vi "MCU_Flashing.vi"(8 "error in (no error)":errorcluster) -> (0 "error in (out)":errorcluster)   [LabVIEW 2024, in "MCU_Flashing.lvlib"]
doc: "This template is for the Queued Message Handler design pattern.\n\nThe Event Handling Loop generates messages based on user interface actions.\n\nThe Message Handling Loop processes messages generated by the Event Handling Loop, or by other messages. The messages are string values, so new messages can be added easily to the Message Cases case structure in the Message Handling Loop. Each message cluster can also provide an optional value for Message Data, which is a variant that can be converted to whatever message-specific data is required."
uses:
  MCU_Flashing.lvlib
  support/MCU_ctrl.ctl
  controls/MCU UI Data.ctl
  PrivateControls/FGV_Queue_Control.ctl
  <vilib>/Utility/error.llb/Error Cluster From Error Code.vi
  <vilib>/ErrorRing/Error Ring.xnode
  support/Message Queue/MCU Message Queue.lvlib
  support/User Event - Stop/MCU User Event - Stop.lvlib
  Launcher/Launcher_DTU.lvlib
panel:
  out "x >= 0?":bool
  in  "MCU Flashing":T1
  in  "Config":string
  in  "DUT":string
  in  "Flash":bool
  out "queue name 2":string
  out "queue name":string
  out "Display <Replace Me>":string
  in  "Init_Neoway":bool
  in  "Exit":bool
  # "These controls have associated \"Value Changed\" events configured in the Event Structure on the diagram.\n\nReplace them (and reconfigure the Event Structure) with the controls you need for your application."
  # "This template is for the Queued Message Handler design pattern.\n\nSee the block diagram for more information on how to use this template."
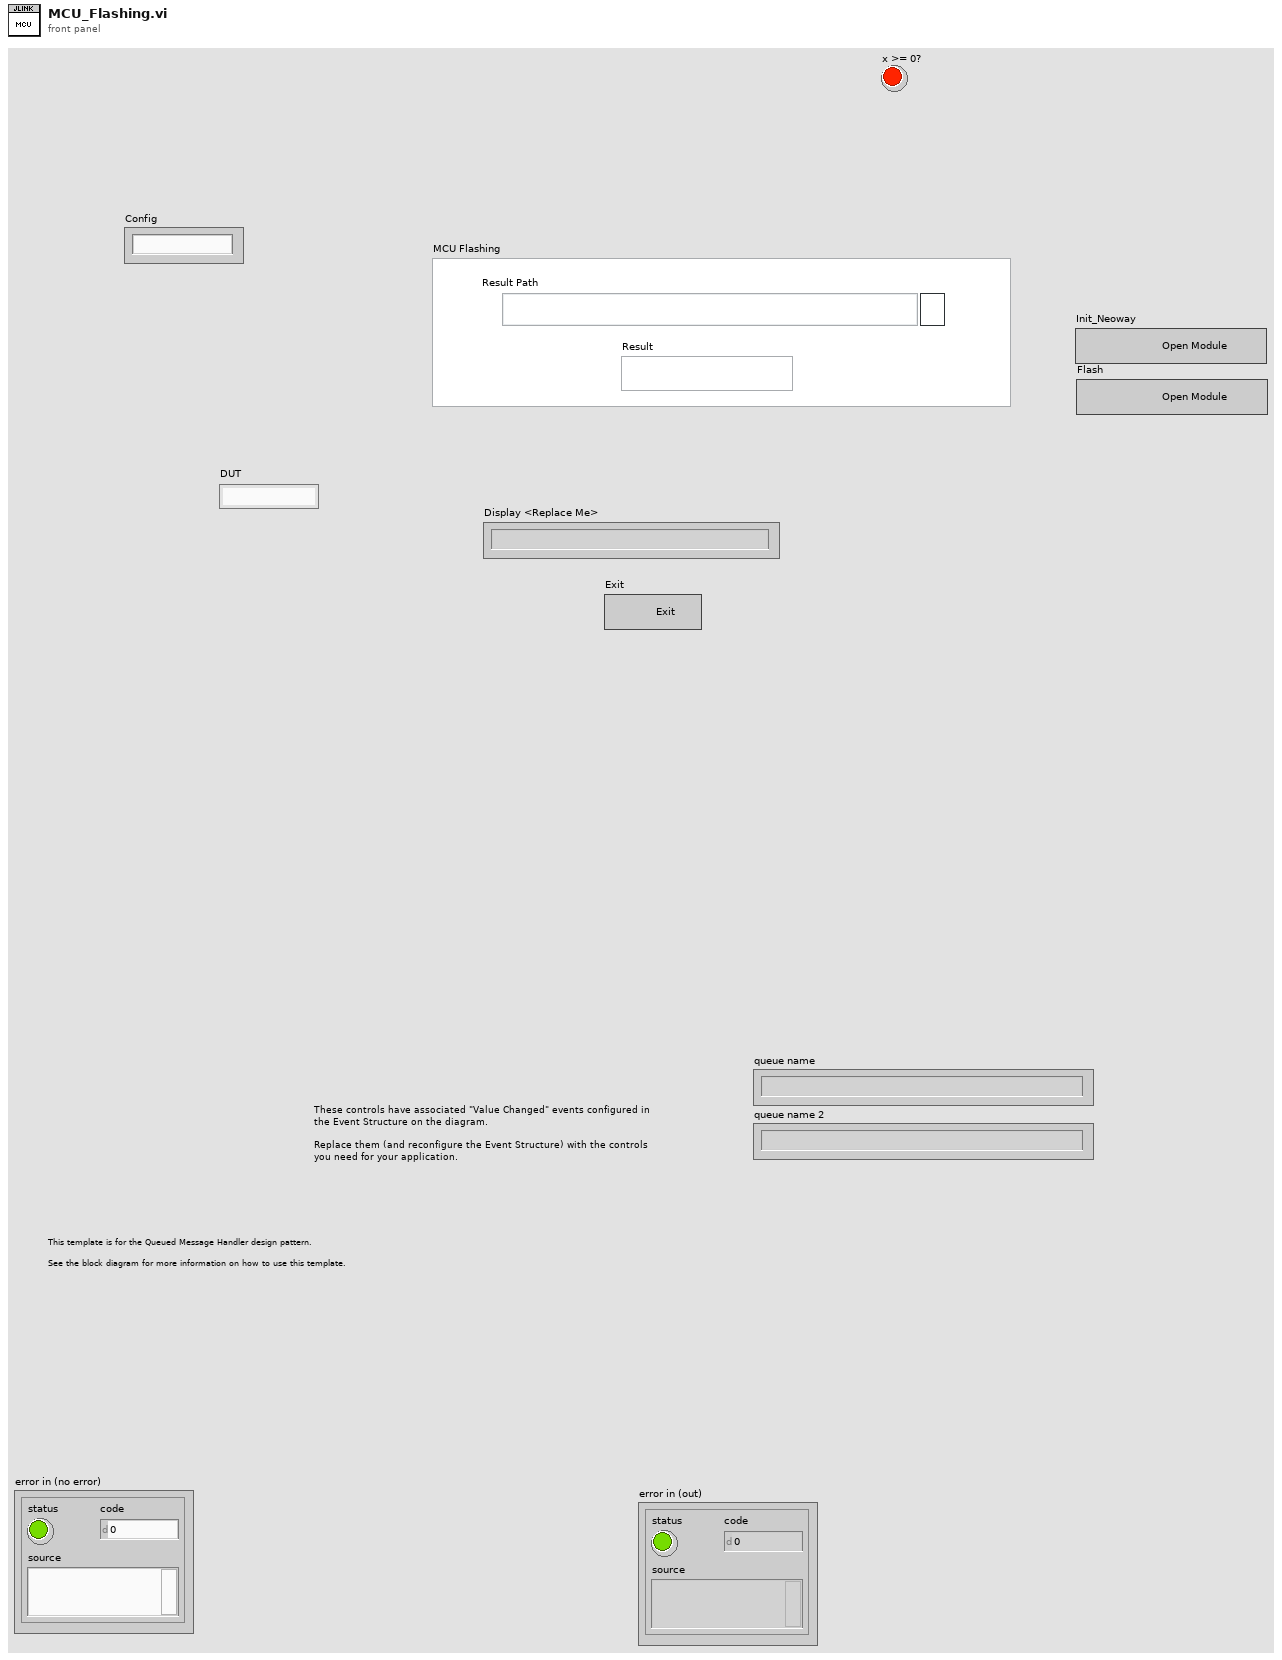
[diagram p1: front panel]
types:
  T1 = typedef "MCU_Flashing.lvlib/MCU_ctrl.ctl" = cluster{"Result Path":path, "Result":string}
  T2 = typedef "MCU_Flashing.lvlib/MCU UI Data.ctl" = cluster{"DUT":string, "Neoway_Q":refnum<queue>, "notifier out":refnum<notifier>, "Config":string, "Neoway Flashing":T1, "Bat file path":path, "Exe path":string, "Flash path":string}
  T3 = typedef "MCU_Flashing.lvlib/FGV_Queue_Control.ctl" = enum16{"Release", "Get", "Set"}
  T4 = typedef "MCU_Flashing.lvlib/MCU Message Queue.lvlib/All Message Queues.ctl" = cluster{"UI":refnum<queue>, "QSM":refnum<queue>}
  T5 = cluster{"Message":string, "Message Data":variant}
  T6 = enum16{"Read", "Write", "All_sections", "All_values", "Remove key&section"}
  T7 = enum16{"open", "replace", "create", "open or create", "replace or create", "replace or create with confirmation"}
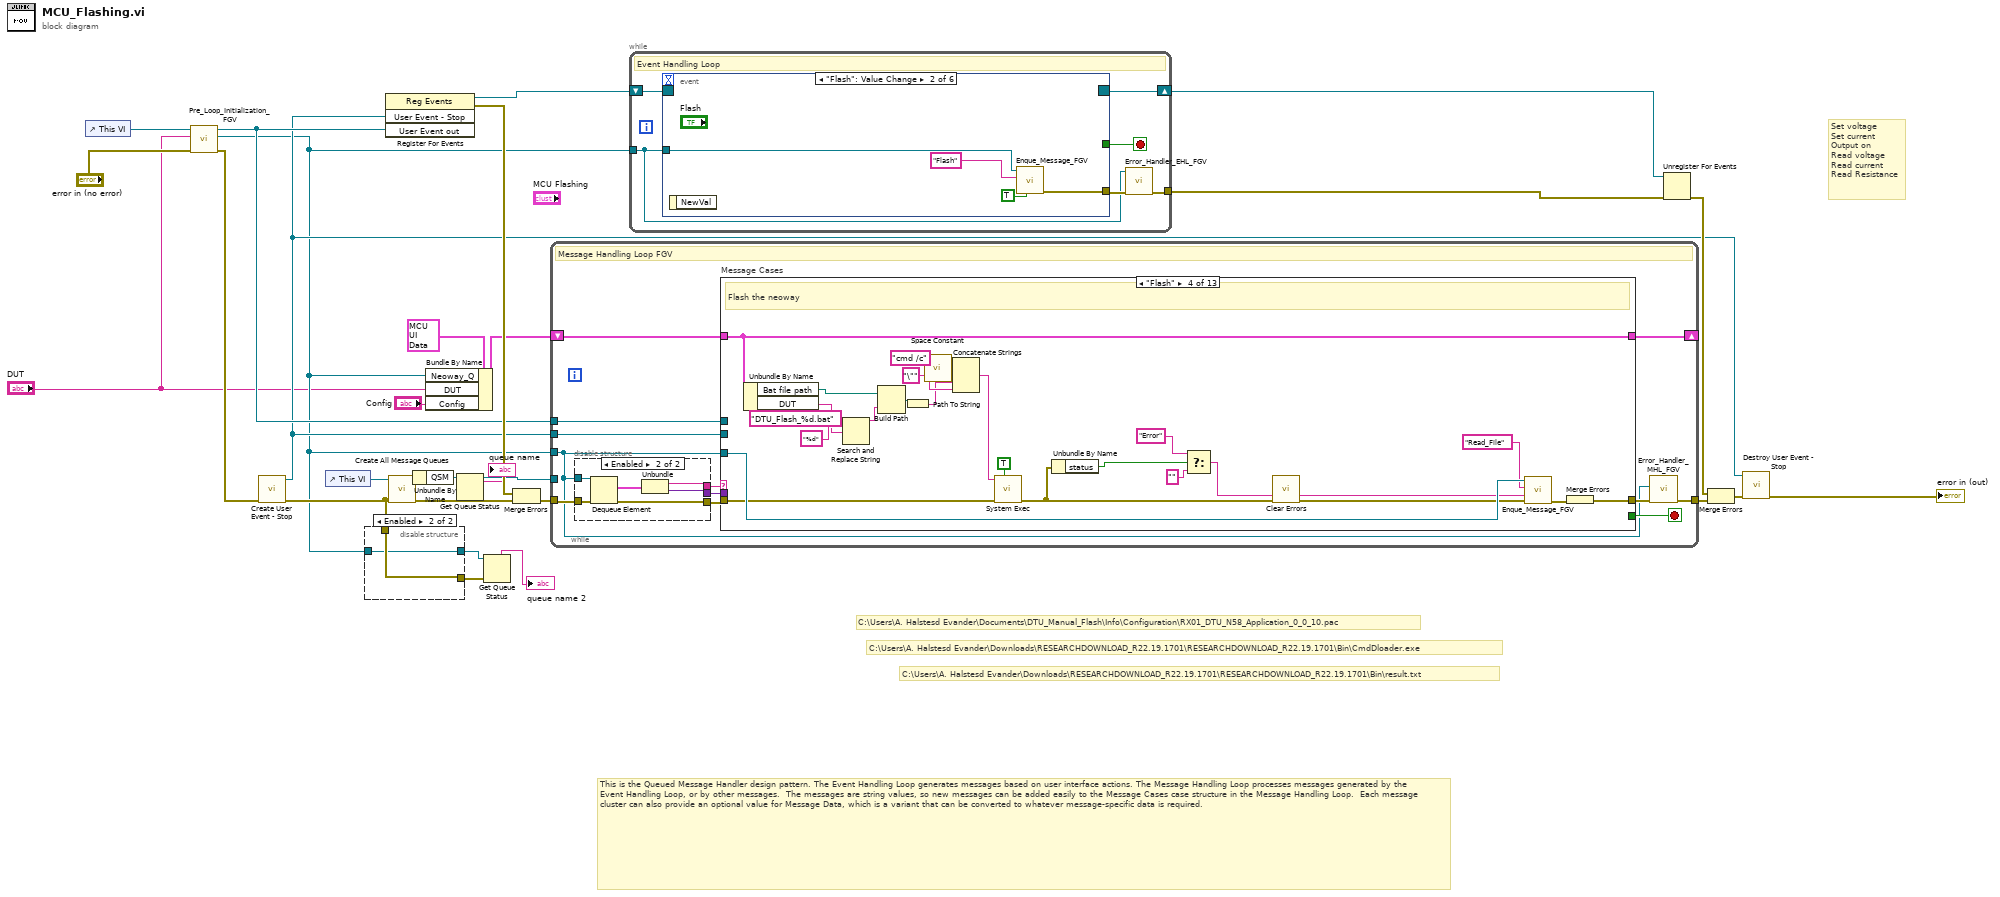
[diagram p0: block diagram]
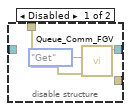
[diagram p2: hidden frame]
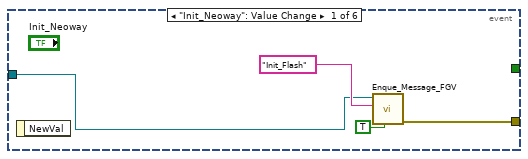
[diagram p3: hidden frame]
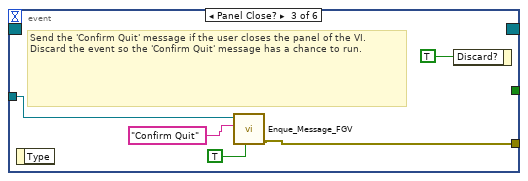
[diagram p4: hidden frame]
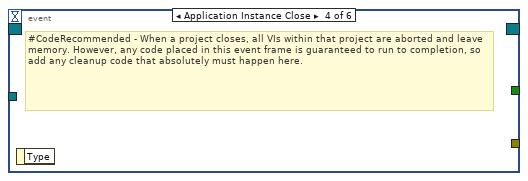
[diagram p5: hidden frame]
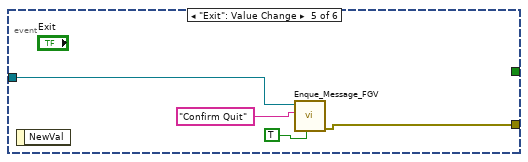
[diagram p6: hidden frame]
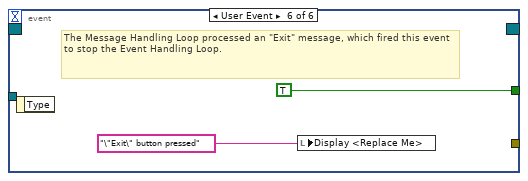
[diagram p7: hidden frame]
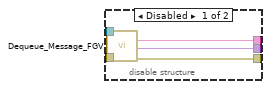
[diagram p8: hidden frame]
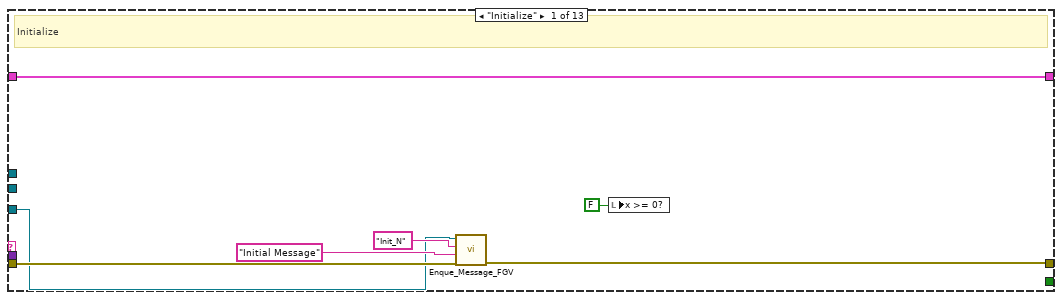
[diagram p9: hidden frame]
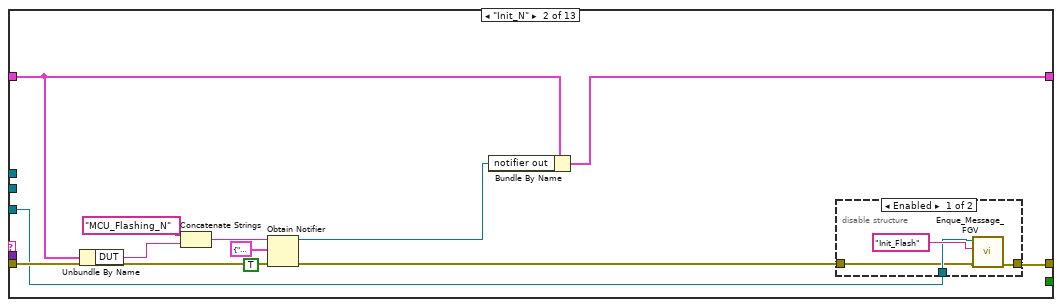
[diagram p10: hidden frame]
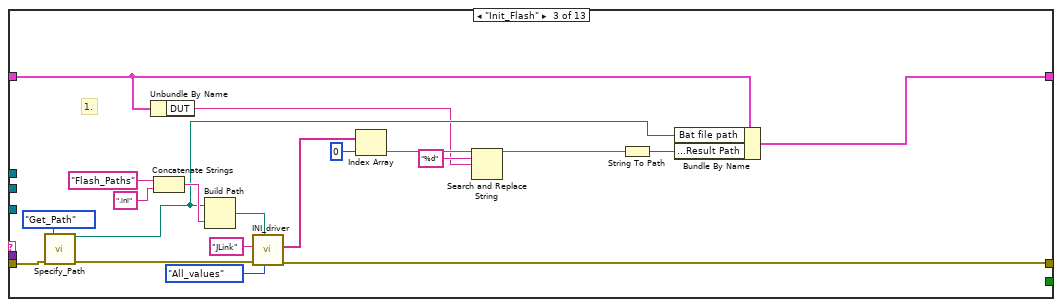
[diagram p12: hidden frame]
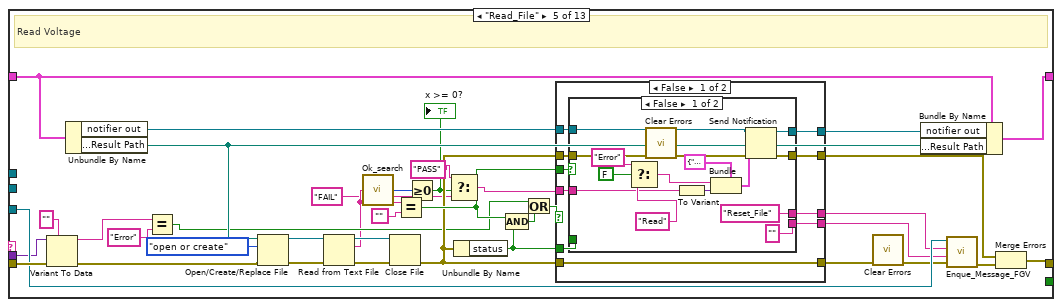
[diagram p13: hidden frame]
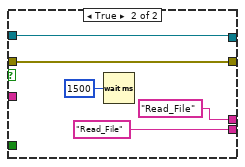
[diagram p14: hidden frame]
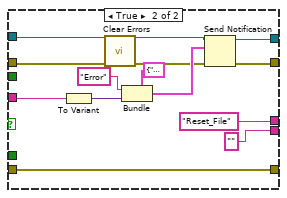
[diagram p15: hidden frame]
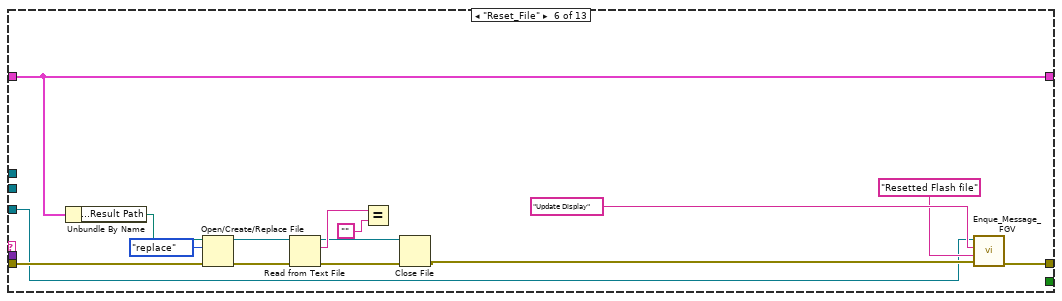
[diagram p16: hidden frame]
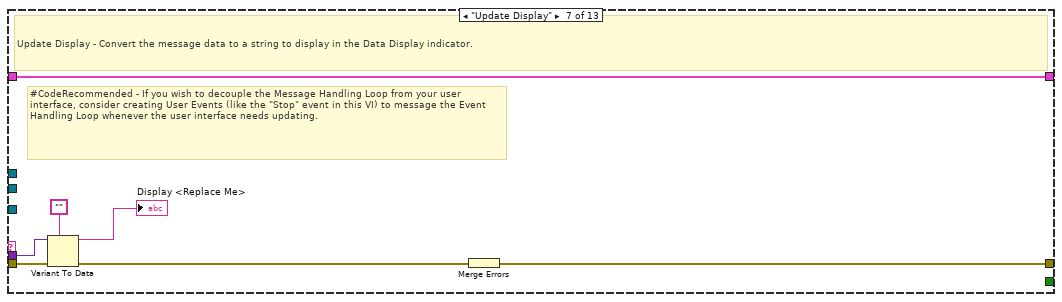
[diagram p17: hidden frame]
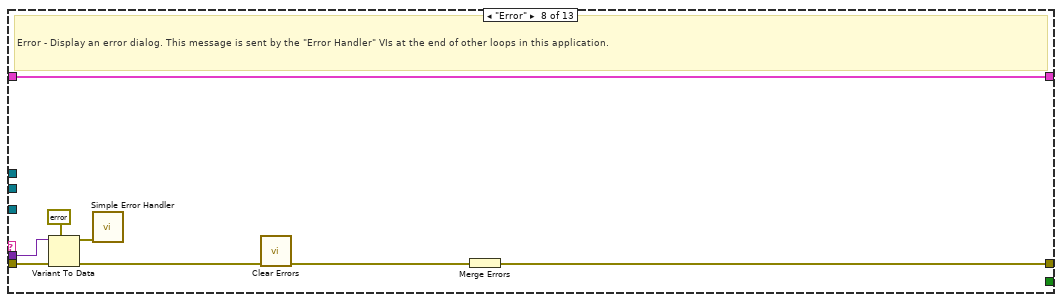
[diagram p18: hidden frame]
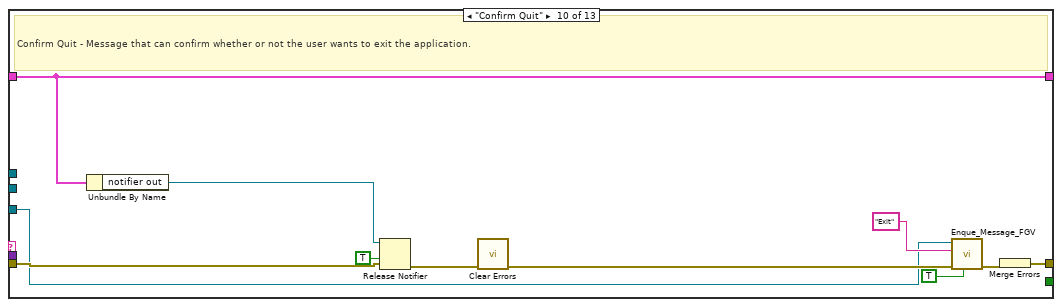
[diagram p20: hidden frame]
diagram:
  # "C:\\Users\\A. Halstesd Evander\\Downloads\\RESEARCHDOWNLOAD_R22.19.1701\\RESEARCHDOWNLOAD_R22.19.1701\\Bin\\result.txt"
  # "C:\\Users\\A. Halstesd Evander\\Downloads\\RESEARCHDOWNLOAD_R22.19.1701\\RESEARCHDOWNLOAD_R22.19.1701\\Bin\\CmdDloader.exe"
  # "C:\\Users\\A. Halstesd Evander\\Documents\\DTU_Manual_Flash\\Info\\Configuration\\RX01_DTU_N58_Application_0_0_10.pac"
  # "Set voltage\nSet current\nOutput on\nRead voltage \nRead current\nRead Resistance"
  # "This is the Queued Message Handler design pattern. The Event Handling Loop generates messages based on user interface actions. The Message Handling Loop processes messages generated by the Event Handling Loop, or by other messages.  The messages are string values, so new messages can be added easily to the Message Cases case structure in the Message Handling Loop.  Each message cluster can also provide an optional value for Message Data, which is a variant that can be converted to whatever message-specific data is required."
  n1 = control-ref of="This VI"() -> (w17:refnum<vi>)
  n2 = call "Pre_Loop_Initialization_FGV.vi"("error in (no error)"="error in (no error)", "DUT"="DUT", "VI in"=w17) -> ("error out"=w15:errorcluster, "queue out"=w3:refnum<queue>, "User Event out"=w7:refnum<user-event>)  [unwired: 6 in]
  n3 = call "Create User Event - Stop.vi"("error in (no error)"=w15) -> ("error out"=w10:errorcluster, "User Event - Stop"=w6:refnum<user-event>)  [unwired: 9 in]
  n4 = control-ref of="This VI"() -> (w13:refnum<vi>)
  n5 = disable-structure shown="Enabled" {
    disable-tunnel: w10 -> [w32 w34]
    disable-tunnel: [w30 w33] -> w9
    disable-tunnel: [_ w34] -> w5
    disable-tunnel: w3 -> [_ w33]
    frame Disabled {
      n6 = call "Queue_Comm_FGV.vi"("error in (no error)"=w32, "Enum"=FGV_Queue_Control."Get") -> ("queue Out"=w30:refnum<queue>)  [unwired: 8 in, 1 out]
    }
    frame Enabled {
    }
  }
  n7 = register-events(w6, w7) -> (reference out=w20:refnum<event-registration>, error out=w18:errorcluster)  [unwired: 2 in]
  n8 = call "Create All Message Queues.vi"("error in (no error)"=w10, "This VI"=w13) -> ("error out"=w29:errorcluster, "Message Queues out"=w28:T4)  [unwired: 8 in]
  n9 = Unbundle By Name(w28) -> ("QSM"=w26:refnum<queue>)
  n10 = Bundle By Name(cluster=T2 {"DUT"="", "Neoway_Q"=refnum, "notifier out"=refnum, "Config"="", "Neoway Flashing"={"Result Path"=path "", "Result"=""}, "Bat file path"=path "", "Exe path"="", "Flash path"=""} ("Data Cluster"), "Neoway_Q"=w3, "DUT"="DUT", "Config"="Config") -> (w4:T2)
  n11 = Get Queue Status(queue=w26) -> (queue out=w12:refnum<queue>, queue name=→"queue name":string)  [unwired: 2 in, 6 out]
  n12 = Get Queue Status(queue=w9, error in (no error)=w5) -> (queue name=→"queue name 2":string)  [unwired: 1 in, 7 out]
  n13 = Merge Errors(w18, w29) -> (w19:errorcluster)
  n14 = while {
    tunnel: w12 -> [_]
    shift-right: [w45] -> _
    shift-left: w4 -> [w46]
    tunnel: w7 -> [w43]
    tunnel: w19 -> [w42]
    tunnel: [w37] -> w27
    tunnel: w6 -> [w36]
    tunnel: w3 -> [w35]
    stop <- w44 stop-if-true
    # "Message Handling Loop FGV"
    n15 = disable-structure shown="Enabled" {
      disable-tunnel: w42 -> [w50 w56]
      disable-tunnel: [w49 w54] -> w41
      disable-tunnel: [w48 w51] -> w40
      disable-tunnel: [w47 w52] -> w39
      disable-tunnel: w35 -> [_ w55]
      frame Disabled {
        n16 = call "Dequeue_Message_FGV.vi"("error in (no error)"=w50) -> ("error out"=w49:errorcluster, "Message Data"=w48:variant, "Message"=w47:string)  [unwired: 8 in]
      }
      frame Enabled {
        n17 = Dequeue Element(queue=w55, error in (no error)=w56) -> (element=w53:T5, error out=w54:errorcluster)  [unwired: 1 in, 2 out]
        n18 = Unbundle(w53) -> ("Message"=w52:string, "Message Data"=w51:variant)
      }
    }
    n19 = case "Message Cases" shown="\"Flash\"" w39 {
      selector: w39 -> [_ _ _ _ _ _ _ _ _ _ _ _ w267]
      tunnel: w41 -> [w59 w75 w100 w121 w161 w219 w224 w234 w236 w245 w250 w258 _]
      tunnel: [w62 w64 w99 w124 w156 w206 w225 w228 w236 w247 w248 w251 w268] -> w38
      tunnel: w46 -> [w63 w73 w83 w120 w159 w218 w226 w233 w235 w242 w249 w253 w269]
      tunnel: [w63 w68 w89 w120 w158 w218 w226 w233 w235 w242 w249 w253 w269] -> w45
      tunnel: [_ _ _ _ _ _ _ _ _ _ _ TRUE _] -> w44
      tunnel: w40 -> [_ _ _ _ w155 _ w223 w232 _ _ _ w260 _]
      tunnel: w43 -> [_ _ _ _ _ _ _ _ _ _ _ w261 _]
      tunnel: w36 -> [_ _ _ _ _ _ _ _ _ _ _ w256 _]
      tunnel: w35 -> [w58 w66 _ w122 w157 w205 _ _ _ w240 _ w252 _]
      frame "Initialize" {
        # "Initialize"
        n20 = call "Enque_Message_FGV.vi"("error in (no error)"=w59, "Message Data"="Initial Message" ("Initial Message"), "Message"="Init_N", "queue in"=w58) -> ("error out"=w62:errorcluster)  [unwired: 7 in]
        n21 = local write "x >= 0?"(FALSE ("x >= 0?")) -> ()
      }
      frame "Init_N" {
        n22 = Unbundle By Name(w73) -> ("DUT"=w72:string)
        n23 = Concatenate Strings("MCU_Flashing_N", w72) -> (w71:string)
        n24 = Obtain Notifier(name (unnamed)=w71, notification data type=T5 {"Message"="", "Message Data"=variant} ("notification"), create if not found? (T)=TRUE, error in (no error)=w75) -> (notifier out=w67:refnum<notifier>, error out=w65:errorcluster)  [unwired: 1 out]
        n25 = Bundle By Name(cluster=w73, "notifier out"=w67) -> (w68:T2)
        n26 = disable-structure shown="Enabled" {
          disable-tunnel: w66 -> [w78 _]
          disable-tunnel: w65 -> [w77 w80]
          disable-tunnel: [w76 w80] -> w64
          frame Enabled {
            n27 = call "Enque_Message_FGV.vi"("error in (no error)"=w77, "Message"="Init_Flash", "queue in"=w78) -> ("error out"=w76:errorcluster)  [unwired: 8 in]
          }
          frame Disabled {
          }
        }
      }
      frame "Init_Flash" {
        # "1."
        n28 = call "Specify_Path.vi"("Path_Enum"=enum16{"Find_Path", "Get_Path"}."Get_Path", "error in (no error)"=w100) -> ("Configurations"=w86:path, "error out"=w94:errorcluster)  [unwired: 6 in, 6 out]
        n29 = Unbundle By Name(w83) -> ("DUT"=w82:string)
        n30 = Concatenate Strings("Flash_Paths" ("string"), ".ini" ("string")) -> (w96:string)
        n31 = Build Path(base path=w86, name or relative path=w96) -> (appended path=w95:path)
        n32 = call "INI_driver.vi"("Enum"=T6."All_values", "instrument file path"=w95, "error in (no error)"=w94, "Section"="JLink") -> ("error out"=w99:errorcluster, "Values out"=w92:string[])  [unwired: 4 in, 2 out]
        n33 = Index Array(array=w92, index=0) -> (element=w84:string)
        n34 = Search and Replace String(input string=w84, search string="%d", replace string=w82) -> (result string=w81:string)  [unwired: 5 in, 3 out]
        n35 = String To Path(string=w81) -> (path=w87:path)
        n36 = Bundle By Name(cluster=w83, "Bat file path"=w86, "Neoway Flashing.Result Path"=w87) -> (w89:T2)
      }
      frame "Flash" {
        w115 = "\"" ("string")
        # "Flash the neoway"
        n37 = Unbundle By Name(w120) -> ("Bat file path"=w119:path, "DUT"=w102:string)
        n38 = Search and Replace String(input string="DTU_Flash_%d.bat", search string="%d", replace string=w102) -> (result string=w101:string)  [unwired: 5 in, 3 out]
        n39 = Build Path(base path=w119, name or relative path=w101) -> (appended path=w118:path)
        n40 = Path To String(path=w118) -> (string=w114:string)
        n41 = call <vilib>:"Space Constant.vi"() -> ("String"=w116:string)
        n42 = Concatenate Strings("cmd /c", w116, w115, w114, w115) -> (w113:string)
        n43 = call <vilib>:"System Exec.vi"("wait until completion? (T)"=TRUE, "error in (no error)"=w121, "command line"=w113) -> ("error out"=w112:errorcluster)  [unwired: 5 in, 3 out]
        n44 = Unbundle By Name(w112) -> ("status"=w109:bool)
        n45 = Select(t="Error" ("\"Do Something\" button pressed"), s=w109, f="" ("\"Do Something\" button pressed")) -> (s? t:f=w107:string)
        n46 = call <vilib>:"Clear Errors.vi"("error in (no error)"=w112) -> ("error out"=w106:errorcluster)  [unwired: 5 in, 1 out]
        n47 = call "Enque_Message_FGV.vi"("error in (no error)"=w106, "Message Data"=w107, "Message"="Read_File", "queue in"=w122) -> ("error out"=w123:errorcluster)  [unwired: 7 in]
        n48 = Merge Errors(w123) -> (w124:errorcluster)
      }
      frame "Read_File" {
        # "Read Voltage"
        n49 = Variant To Data(error in=w161, type="", Variant=w155) -> (data=w152:string, error out=w151:errorcluster)
        n50 = Unbundle By Name(w159) -> ("notifier out"=w142:refnum<notifier>, "Neoway Flashing.Result Path"=w145:path)
        n51 = Equal?(x=w152, y="Error" ("\"Do Something\" button pressed")) -> (x = y?=w134:bool)
        n52 = Open/Create/Replace File(file path (use dialog)=w145, error in=w151, operation (0:open)=T7."open or create") -> (refnum out=w148:refnum<file>, error out=w150:errorcluster)  [unwired: 3 in, 1 out]
        n53 = Read from Text File(file (use dialog)=w148, error in=w150) -> (refnum out=w146:refnum<file>, text=w131:string, error out=w149:errorcluster)  [unwired: 2 in, 1 out]
        n54 = call "Ok_search.vi"("Display"=w131) -> ("index of element"=w130:i32)
        n55 = Close File(refnum=w146, error in=w149) -> (error out=w136:errorcluster)  [unwired: 1 out]
        n56 = Equal?(x=w131, y="") -> (x = y?=w139:bool)
        n57 = Greater Or Equal To 0?(x=w130) -> (x >= 0?=w129:bool)
        "x >= 0?" <- w129
        n58 = Select(t="PASS", s=w129, f="FAIL") -> (s? t:f=w126:string)
        n59 = Unbundle By Name(w136) -> ("status"=w140:bool)
        n60 = Compound Arithmetic op=AND(w139, w140) -> (w133:bool)
        n61 = Or(x=w134, y=w133) -> (x .or. y?=w132:bool)
        n62 = case shown="False" w132 {
          tunnel: w136 -> [w171 w196]
          tunnel: [w170 w197] -> w143
          tunnel: w142 -> [w169 w199]
          tunnel: [w168 w198] -> w141
          tunnel: w126 -> [w167 w194]
          tunnel: w140 -> [w166 _]
          tunnel: w139 -> [w165 _]
          tunnel: [w164 "Reset_File" ("Message")] -> w138
          tunnel: [w163 "" ("\"Do Something\" button pressed")] -> w137
          tunnel: w136 -> [w162 w204]
          tunnel: [w162 w204] -> w135
          frame False {
            n63 = case shown="False" w165 {
              tunnel: w171 -> [w180 w191]
              tunnel: [w178 w191] -> w170
              tunnel: w169 -> [w177 w190]
              tunnel: [w176 w190] -> w168
              tunnel: w167 -> [w175 _]
              tunnel: w166 -> [_ _]
              tunnel: ["Reset_File" ("Message") "Read_File" ("Message")] -> w164
              tunnel: ["" ("\"Do Something\" button pressed") "Read_File" ("\"Do Something\" button pressed")] -> w163
              frame False {
                n64 = Select(t="Error" ("f"), s=FALSE, f="Read" ("Message")) -> (s? t:f=w186:string)
                n65 = call <vilib>:"Clear Errors.vi"("error in (no error)"=w180) -> ("error out"=w179:errorcluster)  [unwired: 5 in, 1 out]
                n66 = To Variant(anything=w175) -> (Variant=w185:variant)
                n67 = Bundle(cluster=T5 {"Message"="", "Message Data"=variant} ("notification"), "Message"=w186, "Message Data"=w185) -> (w184:T5)
                n68 = Send Notification(notification=w184, notifier=w177, error in (no error)=w179) -> (notifier out=w176:refnum<notifier>, error out=w178:errorcluster)
              }
              frame True {
                n69 = Wait (ms)(milliseconds to wait=u32 1500) -> ()  [unwired: 1 out]
              }
            }
          }
          frame True {
            n70 = To Variant(anything=w194) -> (Variant=w203:variant)
            n71 = call <vilib>:"Clear Errors.vi"("error in (no error)"=w196) -> ("error out"=w200:errorcluster)  [unwired: 5 in, 1 out]
            n72 = Bundle(cluster=T5 {"Message"="", "Message Data"=variant} ("notification"), "Message"="Error" ("f"), "Message Data"=w203) -> (w202:T5)
            n73 = Send Notification(notification=w202, notifier=w199, error in (no error)=w200) -> (notifier out=w198:refnum<notifier>, error out=w197:errorcluster)
          }
        }
        n74 = call <vilib>:"Clear Errors.vi"("error in (no error)"=w135) -> ("error out"=w144:errorcluster)  [unwired: 5 in, 1 out]
        n75 = Bundle By Name(cluster=w159, "notifier out"=w141, "Neoway Flashing.Result Path"=w145) -> (w158:T2)
        n76 = call "Enque_Message_FGV.vi"("error in (no error)"=w144, "Message Data"=w137, "Message"=w138, "queue in"=w157) -> ("error out"=w160:errorcluster)  [unwired: 7 in]
        n77 = Merge Errors(w143, w160) -> (w156:errorcluster)
      }
      frame "Reset_File" {
        n78 = Unbundle By Name(w218) -> ("Neoway Flashing.Result Path"=w216:path)
        n79 = Open/Create/Replace File(file path (use dialog)=w216, error in=w219, operation (0:open)=T7."replace") -> (refnum out=w213:refnum<file>, error out=w217:errorcluster)  [unwired: 3 in, 1 out]
        n80 = Read from Text File(file (use dialog)=w213, error in=w217) -> (refnum out=w210:refnum<file>, text=w211:string, error out=w214:errorcluster)  [unwired: 2 in, 1 out]
        n81 = Equal?(x=w211, y="") -> ()  [unwired: 1 out]
        n82 = Close File(refnum=w210, error in=w214) -> (error out=w207:errorcluster)  [unwired: 1 out]
        n83 = call "Enque_Message_FGV.vi"("error in (no error)"=w207, "Message Data"="Resetted Flash file" ("\"Do Something\" button pressed"), "Message"="Update Display", "queue in"=w205) -> ("error out"=w206:errorcluster)  [unwired: 7 in]
      }
      frame "Update Display" {
        # "#CodeRecommended - If you wish to decouple the Message Handling Loop from your user interface, consider creating User Events (like the \"Stop\" event in this VI) to message the Event Handling Loop whenever the user interface needs updating."
        # "Update Display - Convert the message data to a string to display in the Data Display indicator."
        n84 = Variant To Data(error in=w224, type="", Variant=w223) -> (data=→"Display <Replace Me>":string, error out=w221:errorcluster)
        n85 = Merge Errors(w221) -> (w225:errorcluster)
      }
      frame "Error" {
        # "Error - Display an error dialog. This message is sent by the \"Error Handler\" VIs at the end of other loops in this application."
        n86 = Variant To Data(error in=w234, type=errorcluster {"status"=FALSE, "code"=0, "source"=""} ("error constant"), Variant=w232) -> (data=w230:errorcluster, error out=w229:errorcluster)
        n87 = call <vilib>:"Simple Error Handler.vi"("error in (no error)"=w230) -> ()  [unwired: 4 in, 5 out]
        n88 = call <vilib>:"Clear Errors.vi"("error in (no error)"=w229) -> ("error out"=w227:errorcluster)  [unwired: 5 in, 1 out]
        n89 = Merge Errors(w227) -> (w228:errorcluster)
      }
      frame "Reset" {
      }
      frame "Confirm Quit" {
        # "Confirm Quit - Message that can confirm whether or not the user wants to exit the application."
        n90 = Unbundle By Name(w242) -> ("notifier out"=w238:refnum<notifier>)
        n91 = Release Notifier(notifier=w238, force destroy? (F)=TRUE, error in (no error)=w245) -> (error out=w239:errorcluster)  [unwired: 2 out]
        n92 = call <vilib>:"Clear Errors.vi"("error in (no error)"=w239) -> ("error out"=w241:errorcluster)  [unwired: 5 in, 1 out]
        n93 = call "Enque_Message_FGV.vi"("Priority"=TRUE ("Priority Message? (F)"), "error in (no error)"=w241, "Message"="Exit", "queue in"=w240) -> ("error out"=w246:errorcluster)  [unwired: 7 in]
        n94 = Merge Errors(w246) -> (w247:errorcluster)
      }
      frame "---Copy This Frame---" {
        # "Duplicate this frame when creating new messages.  Change this comment in the duplicated frame to describe this message."
        n95 = Merge Errors(w250) -> (w248:errorcluster)
      }
      frame "Exit" {
        # "Stop the VI"
        # "Release the message queue reference"
        # "Exit - Exit the application."
        n96 = disable-structure shown="Disabled" {
          disable-tunnel: w260 -> [w264 _]
          frame Disabled {
            n97 = Variant To Data(type=errorcluster {"status"=FALSE, "code"=0, "source"=""} ("error constant"), Variant=w264) -> (data=w265:errorcluster)  [unwired: 1 in, 1 out]
            n98 = call <vilib>:"Simple Error Handler.vi"("error in (no error)"=w265) -> ()  [unwired: 4 in, 5 out]
          }
          frame Enabled {
          }
        }
        n99 = call "Queue_Comm_FGV.vi"("error in (no error)"=w258, "Enum"=FGV_Queue_Control."Release", "queue in"=w252) -> ("error Out"=w257:errorcluster)  [unwired: 7 in, 1 out]
        n100 = call "Fire User Event - Stop.vi"("User Event - Stop"=w256) -> ("error out"=w254:errorcluster)  [unwired: 10 in]
        n101 = call "Fire User Event - Stop.vi"("User Event - Stop"=w261) -> ("error out"=w255:errorcluster)  [unwired: 10 in]
        n102 = Merge Errors(w255, w254, w257) -> (w262:errorcluster)
        n103 = call <vilib>:"Clear Errors.vi"("error in (no error)"=w262) -> ("error out"=w251:errorcluster)  [unwired: 5 in, 1 out]
      }
      frame Default {
        # "'Default' case only runs if there is a message that isn't defined in any of the other cases.  Output a programming error."
        n104 = xnode "Error Ring"("parameter 0"=w267) -> ("error out"=w268:errorcluster)
      }
    }
    n105 = call "Error_Handler_MHL_FGV.vi"("error in (no error)"=w38, "queue in"=w35) -> ("error Out"=w37:errorcluster)  [unwired: 9 in]
  }
  n106 = while {
    shift-right: [w281] -> w23
    shift-left: w20 -> [w282]
    tunnel: [w278] -> w21
    tunnel: w3 -> [w277]
    stop <- w280 stop-if-true
    # "Event Handling Loop"
    n107 = event shown="[1] \"Flash\": Value Change" {
      selector: w282 -> [_ _ _ _ _ _]
      dyn-events: [_ _ _ _ _ _] -> w281
      timeout: _ -> [_ _ _ _ _ _]
      tunnel: [_ _ _ _ _ TRUE ("Discard?")] -> w280
      tunnel: [w285 w289 w294 _ w299 _] -> w279
      tunnel: w277 -> [w283 w287 w291 _ w296 _]
      event "Init_Neoway": Value Change {
        n108 = event-data() -> ()  [unwired: 1 in, 1 out]
        n109 = call "Enque_Message_FGV.vi"("Priority"=TRUE ("Priority Message? (F)"), "Message"="Init_Flash", "queue in"=w283) -> ("error out"=w285:errorcluster)  [unwired: 8 in]
      }
      event "Flash": Value Change {
        n110 = event-data() -> ()  [unwired: 1 in, 1 out]
        n111 = call "Enque_Message_FGV.vi"("Priority"=TRUE ("Priority Message? (F)"), "Message"="Flash", "queue in"=w287) -> ("error out"=w289:errorcluster)  [unwired: 8 in]
      }
      event Panel Close? {
        # "Send the 'Confirm Quit' message if the user closes the panel of the VI. Discard the event so the 'Confirm Quit' message has a chance to run."
        n112 = event-data() -> ()  [unwired: 1 in, 1 out]
        n113 = call "Enque_Message_FGV.vi"("Priority"=TRUE ("Priority Message? (F)"), "Message"="Confirm Quit", "queue in"=w291) -> ("error out"=w294:errorcluster)  [unwired: 8 in]
        n114 = event-data("Discard?"=TRUE) -> ()  [unwired: 1 in, 1 out]
      }
      event Application Instance Close {
        # "#CodeRecommended - When a project closes, all VIs within that project are aborted and leave memory. However, any code placed in this event frame is guaranteed to run to completion, so add any cleanup code that absolutely must happen here."
        n115 = event-data() -> ()  [unwired: 1 in, 1 out]
      }
      event "Exit": Value Change {
        n116 = event-data() -> ()  [unwired: 1 in, 1 out]
        n117 = call "Enque_Message_FGV.vi"("Priority"=TRUE ("Priority Message? (F)"), "Message"="Confirm Quit", "queue in"=w296) -> ("error out"=w299:errorcluster)  [unwired: 8 in]
      }
      event User Event {
        # "The Message Handling Loop processed an \"Exit\" message, which fired this event to stop the Event Handling Loop."
        n118 = event-data() -> ()  [unwired: 1 in, 1 out]
        n119 = local write "Display <Replace Me>"("\"Exit\" button pressed" ("VI Stopped")) -> ()
      }
    }
    n120 = call "Error_Handler_EHL_FGV.vi"("error in (no error)"=w279, "queue in"=w277) -> ("error Out"=w278:errorcluster)  [unwired: 9 in]
  }
  n121 = Unregister For Events(event registration refnum=w23, error in=w21) -> (error out=w24:errorcluster)
  n122 = Merge Errors(w24, w27) -> (w25:errorcluster)
  n123 = call "Destroy User Event - Stop.vi"("error in (no error)"=w25, "User Event - Stop"=w6) -> ("error out"=→"error in (out)":errorcluster)  [unwired: 9 in]
